vi "constructCommand_Relay.vi"(6 "Time Stamp":timestamp, 8 "error in (no error)":errorcluster, 9 "svValue":variant, 10 "svArrayIndex":i32, 11 "DataListenerThisComponent in":refnum<class "DataListenerThisComponent.lvclass">) -> (0 "error out":errorcluster, 1 "validIsTrue":bool, 3 "DataListenerThisComponent out":refnum<class "DataListenerThisComponent.lvclass">)   [LabVIEW 2015]
doc: "Turns received shared variable information (from SubDataSVs) into commands (for the Command SV)."
uses:
  ComponentTemplateCore/ComponentModel/ComponentModel/DataListener/DataListener.lvclass
  DataListenerThisComponent.lvclass
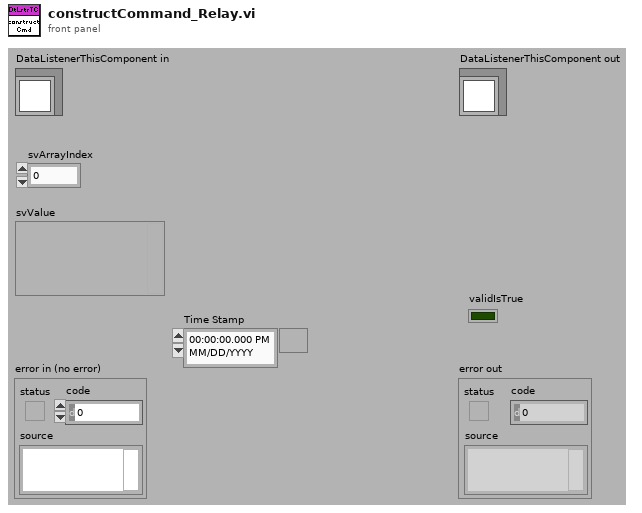
[diagram p1: front panel]
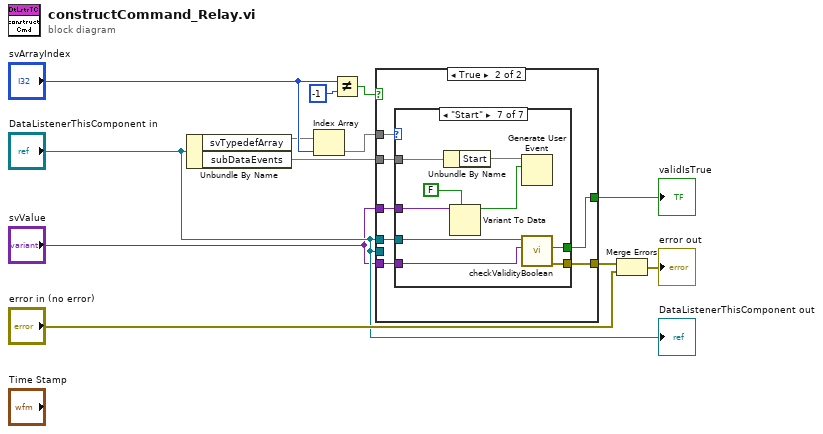
[diagram p0: block diagram]
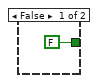
[diagram p2: hidden frame]
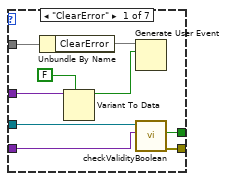
[diagram p3: hidden frame]
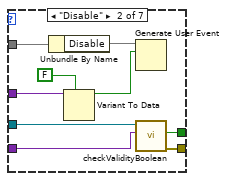
[diagram p4: hidden frame]
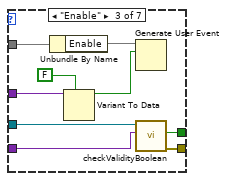
[diagram p5: hidden frame]
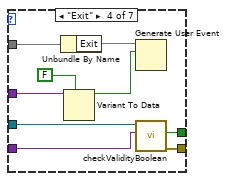
[diagram p6: hidden frame]
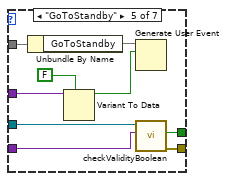
[diagram p7: hidden frame]
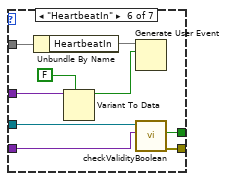
[diagram p8: hidden frame]
diagram:
  n1 = Unbundle By Name("DataListenerThisComponent in") -> ("svTypedefArray"=w9, "subDataEvents"=w1)
  n2 = Index Array(array=w9, index="svArrayIndex") -> (element=w7)
  n3 = Not Equal?(x="svArrayIndex", y=-1) -> (x != y?=w5:bool)
  n4 = case shown="True" w5 {
    tunnel: "svValue" -> [_ w17]
    tunnel: [_ w20] -> w8
    tunnel: w7 -> [_ w19]
    tunnel: [FALSE w14] -> w2
    tunnel: "DataListenerThisComponent in" -> [_ _]
    tunnel: w1 -> [_ w18]
    tunnel: "DataListenerThisComponent in" -> [_ w16]
    tunnel: "svValue" -> [_ w15]
    frame False {
    }
    frame True {
      n5 = case shown="\"Start\"" w19 {
        tunnel: w17 -> [w27 w36 w45 w54 w63 w72 w81]
        tunnel: [w22 w31 w40 w49 w58 w67 w76] -> w20
        tunnel: w18 -> [w29 w38 w47 w56 w65 w74 w83]
        tunnel: w16 -> [w24 w33 w42 w51 w60 w69 w78]
        tunnel: w15 -> [w23 w32 w41 w50 w59 w68 w77]
        tunnel: [w21 w30 w39 w48 w57 w66 w75] -> w14
        frame "ClearError" {
          n6 = Unbundle By Name(w29) -> ("ClearError"=w28)
          n7 = Variant To Data(type=FALSE ("event data"), Variant=w27) -> (data=w25:bool)  [unwired: 1 in, 1 out]
          n8 = Generate User Event(user event=w28, event data cluster=w25) -> ()  [unwired: 2 in, 2 out]
          n9 = call "checkValidityBoolean.vi"("svValue"=w23, "DataListener in"=w24) -> ("error out"=w22:errorcluster, "validIsTrue"=w21:bool)  [unwired: 7 in, 1 out]
        }
        frame "Disable" {
          n10 = Unbundle By Name(w38) -> ("Disable"=w37)
          n11 = Variant To Data(type=FALSE ("event data"), Variant=w36) -> (data=w34:bool)  [unwired: 1 in, 1 out]
          n12 = Generate User Event(user event=w37, event data cluster=w34) -> ()  [unwired: 2 in, 2 out]
          n13 = call "checkValidityBoolean.vi"("svValue"=w32, "DataListener in"=w33) -> ("error out"=w31:errorcluster, "validIsTrue"=w30:bool)  [unwired: 7 in, 1 out]
        }
        frame "Enable" {
          n14 = Unbundle By Name(w47) -> ("Enable"=w46)
          n15 = Variant To Data(type=FALSE ("event data"), Variant=w45) -> (data=w43:bool)  [unwired: 1 in, 1 out]
          n16 = Generate User Event(user event=w46, event data cluster=w43) -> ()  [unwired: 2 in, 2 out]
          n17 = call "checkValidityBoolean.vi"("svValue"=w41, "DataListener in"=w42) -> ("error out"=w40:errorcluster, "validIsTrue"=w39:bool)  [unwired: 7 in, 1 out]
        }
        frame "Exit" {
          n18 = Unbundle By Name(w56) -> ("Exit"=w55)
          n19 = Variant To Data(type=FALSE ("event data"), Variant=w54) -> (data=w52:bool)  [unwired: 1 in, 1 out]
          n20 = Generate User Event(user event=w55, event data cluster=w52) -> ()  [unwired: 2 in, 2 out]
          n21 = call "checkValidityBoolean.vi"("svValue"=w50, "DataListener in"=w51) -> ("error out"=w49:errorcluster, "validIsTrue"=w48:bool)  [unwired: 7 in, 1 out]
        }
        frame "GoToStandby" {
          n22 = Unbundle By Name(w65) -> ("GoToStandby"=w64)
          n23 = Variant To Data(type=FALSE ("event data"), Variant=w63) -> (data=w61:bool)  [unwired: 1 in, 1 out]
          n24 = Generate User Event(user event=w64, event data cluster=w61) -> ()  [unwired: 2 in, 2 out]
          n25 = call "checkValidityBoolean.vi"("svValue"=w59, "DataListener in"=w60) -> ("error out"=w58:errorcluster, "validIsTrue"=w57:bool)  [unwired: 7 in, 1 out]
        }
        frame "HeartbeatIn" {
          n26 = Unbundle By Name(w74) -> ("HeartbeatIn"=w73)
          n27 = Variant To Data(type=FALSE ("event data"), Variant=w72) -> (data=w70:bool)  [unwired: 1 in, 1 out]
          n28 = Generate User Event(user event=w73, event data cluster=w70) -> ()  [unwired: 2 in, 2 out]
          n29 = call "checkValidityBoolean.vi"("svValue"=w68, "DataListener in"=w69) -> ("error out"=w67:errorcluster, "validIsTrue"=w66:bool)  [unwired: 7 in, 1 out]
        }
        frame "Start" {
          n30 = Unbundle By Name(w83) -> ("Start"=w82)
          n31 = Variant To Data(type=FALSE ("event data"), Variant=w81) -> (data=w79:bool)  [unwired: 1 in, 1 out]
          n32 = Generate User Event(user event=w82, event data cluster=w79) -> ()  [unwired: 2 in, 2 out]
          n33 = call "checkValidityBoolean.vi"("svValue"=w77, "DataListener in"=w78) -> ("error out"=w76:errorcluster, "validIsTrue"=w75:bool)  [unwired: 7 in, 1 out]
        }
      }
    }
  }
  "validIsTrue" <- w2
  n34 = Merge Errors(w8, "error in (no error)") -> (→"error out":errorcluster)
  "DataListenerThisComponent out" <- "DataListenerThisComponent in"
